vi "Get EOF String.vi"(8 "error in (no error)":errorcluster, 11 "VISA resource name":refnum<visa-resource-name>) -> (0 "error out":errorcluster, 1 "2nd Character":i32, 2 "1st Character":i32, 3 "VISA resource name out":refnum<visa-resource-name>)   [LabVIEW 2011, in "Fluke 5XXX Series Multicalibrators.lvlib"]
doc: "This VI returns the End-Of-File character string.\n\nNote:\n\nThis VI is available only for instrument models 5700A and 5720A."
uses:
  Fluke 5XXX Series Multicalibrators.lvlib
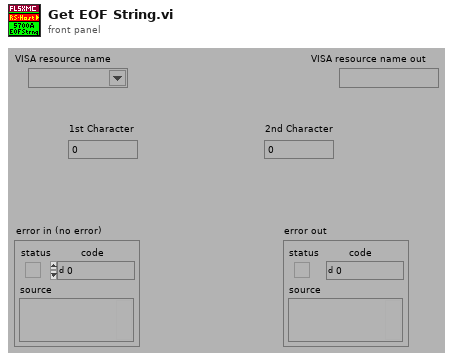
[diagram p1: front panel]
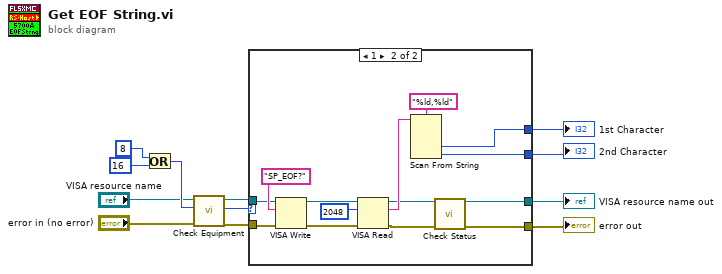
[diagram p0: block diagram]
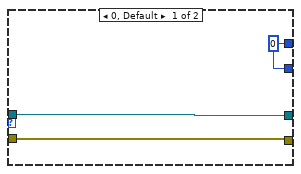
[diagram p2: hidden frame]
diagram:
  n1 = Or(x=8 ("Numeric"), y=16 ("Numeric")) -> (x .or. y?=w10:i32)
  n2 = call "Check Equipment.vi"("error in (no error)"="error in (no error)", "Bit Mask"=w10, "VISA resource name"="VISA resource name") -> ("error out"=w9:errorcluster, "Present?"=w7:u32, "VISA resource name out"=w8:refnum<visa-resource-name>)  [unwired: 6 in]
  n3 = case shown="1" w7 {
    tunnel: [w15 w23] -> w4
    tunnel: [w14 w22] -> w3
    tunnel: w9 -> [w15 w25]
    tunnel: w8 -> [w14 w24]
    tunnel: [w13 w17] -> w2
    tunnel: [w13 w16] -> w1
    frame 0, Default {
      w13 = 0
    }
    frame 1 {
      n4 = VISA Write(VISA resource name=w24, write buffer="SP_EOF?", error in (no error)=w25) -> (VISA resource name out=w28:refnum<visa-resource-name>, error out=w27:errorcluster)  [unwired: 1 out]
      n5 = VISA Read(VISA resource name=w28, byte count=u32 2048 ("byte count (0)"), error in (no error)=w27) -> (VISA resource name out=w18:refnum<visa-resource-name>, read buffer=w20:string, error out=w19:errorcluster)  [unwired: 1 out]
      n6 = Scan From String(format string="%ld,%ld", input string=w20) -> (output 1=w17:i32, output 2=w16:i32)  [unwired: 4 in, 3 out]
      n7 = call "Check Status.vi"("VISA resource name"=w18, "error in (no error)"=w19) -> ("VISA resource name out"=w22:refnum<visa-resource-name>, "error out"=w23:errorcluster)  [unwired: 12 in]
    }
  }
  "1st Character" <- w2
  "2nd Character" <- w1
  "VISA resource name out" <- w3
  "error out" <- w4
